vi "06-QNET_MECHKIT_Sonar.vi"() -> ()   [LabVIEW 2017]
doc: "This VI is to be used with the NI-ELVIS and the QNET-Mechatronic Sensors I module. The objective is to calibrate the Sonar sensor."
uses:
  <vilib>/Simulation/Scripting/Companion Diagram/SimConfigNode/SimParams.ctl
  <vilib>/Simulation/Scripting/Companion Diagram/SimConfigNode/_simSolvers.ctl
  <vilib>/Simulation/Implementation/Shared/SIMSCR Execution Mode.ctl
  <vilib>/Simulation/Param Hierarchy/Typedefs/SIMPH Param Control Actions.ctl
  <vilib>/Simulation/Implementation/Shared/NILVSim_ParamChanged.vi
  <vilib>/Simulation/Implementation/Shared/NILVSIM_BeginStep.vi
  <vilib>/DAQmx/read.llb/DAQmx Read.vi
  <vilib>/DAQmx/read.llb/DAQmx Read (Analog DBL 1Chan 1Samp).vi
  <vilib>/Simulation/SignalDisplay/Implementation/NILVSim Time Waveform.llb/SIM Time Waveform (scalar).vi
  <vilib>/Simulation/Utility/Implementation/SIM Halt.vi
  <vilib>/Simulation/Implementation/Shared/NILVSim_Manager.vi
  <vilib>/Utility/error.llb/Clear Errors.vi
  <vilib>/Simulation/Implementation/Shared/NILVSim_FinalizeModel.vi
  <vilib>/Simulation/Implementation/Shared/SIM Unbundle Sim Info.vi
  <vilib>/Simulation/Implementation/Shared/NILVSim_Initialize.vi
  <vilib>/Analysis/6fits.llb/Linear Fit.vi
  <vilib>/DAQmx/miscellaneous.llb/DAQmx Fill In Error Info.vi
  <vilib>/Simulation/Utility/Implementation/NILVSim Get Time and IsAcceptedStep.vi
  <vilib>/Simulation/Implementation/Shared/SIMSH Read Queue.vi
  <vilib>/Simulation/Implementation/Shared/NILVSim_GetModelError.vi
  <vilib>/Simulation/Implementation/Shared/SIM Bundle Sim Info.vi
  <vilib>/Simulation/Scripting/Companion Diagram/SimConfigNode/SimDog.xnode
  <vilib>/Simulation/Implementation/XNodeFramework/SimXNode/SimX.xnode
  <vilib>/Analysis/NI_AALPro.lvlib
  <vilib>/Simulation/Implementation/Shared/NI_SIM_Implementation.lvlib
panel:
  in  "Sampling Rate (Hz)":dbl=100.0 min=0.0 max=1000.0 step=25.0 format="%.1f"
  in  "Device":tag="Dev1"
  in  "Tab Control":enum32{"Collect Data", "Calibrate Sensor"}(tab)
  out "slope":dbl format="%_3f"
  out "intercept":dbl format="%_3f"
  out "Sonar (V)":waveform(dbl)(graph)
  in  "Target Range (in)":dbl[](array[numeric])
  in  "Sensor Measurement (V)":dbl[](array[numeric])
  out "Sensor Readings":T1(graph)
  out "Sonar (inch) 2":dbl(knob) scale=0.0..20.0
  in  "Offset (in)":dbl
  in  "Calibration Gain (in/V)":dbl
  out "Sonar (inch)":waveform(dbl)(graph)
  in  "stop":bool
  # "QNET-MECHKIT Sonar"
  # "NOTE: Place J9 jumper on \"Sonar\" setting."
  # "1) Move target at different positions.\n2) Enter distance between Sonar and target in \"Target Range (in)\" array.\n3) Enter measured sensor values in \"Sensor Measurement (V)\" array."
  # "Linear curve fitting results:"
  # "Enter gain and offset values for sonar to measure the correct target position\n(e.g. display below should read 8-inches when target is 8-inches away from sonar sensor)."
  # "y = Gain*x + Offset\nwhere\nx is the sensor voltage \ny is the output in inches."
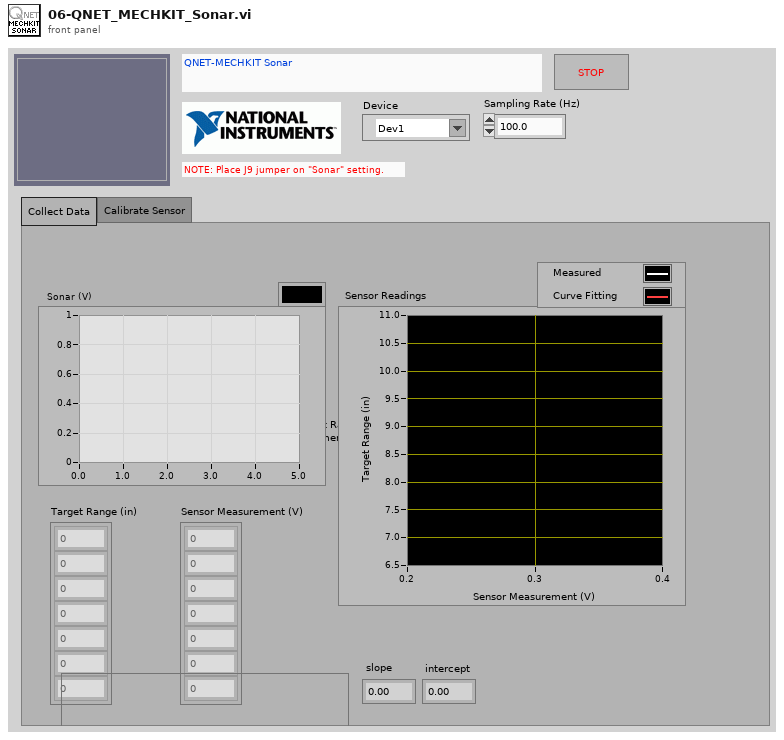
[diagram p1: front panel]
types:
  T1 = cluster{"Sensor Measurement (V)":dbl[], "Best Linear Fit":dbl[]}[]
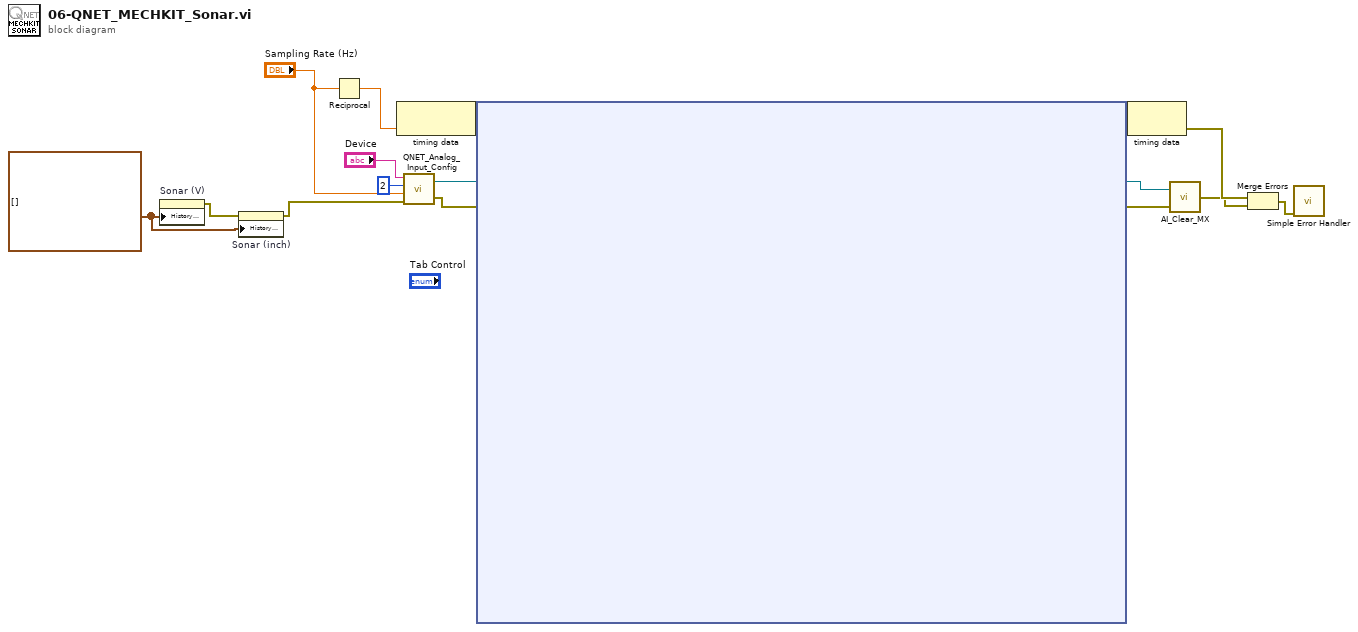
[diagram p0: block diagram]
diagram:
  w1 = waveform(dbl)[] [] ("History Data")
  n1 = property on="Sonar (V)" class="WFChart (strict)"("History Data"=w1) -> (error out=w3:errorcluster)  [unwired: 2 in, 1 out]
  n2 = property on="Sonar (inch)" class="WFChart (strict)"(error in=w3, "History Data"=w1) -> (error out=w2:errorcluster)  [unwired: 1 in, 1 out]
  n3 = Reciprocal(x="Sampling Rate (Hz)") -> (1/x=w8:dbl)
  n4 = node-c288(w8) -> (w16:variant)
  n5 = call "QNET_Analog_Input_Config.vi"("error in"=w2, "sampling rate (Hz)"="Sampling Rate (Hz)", "analog input channel"=u32 2, "dev"="Device") -> ("error out"=w13:errorcluster, "task out"=w12:refnum<k21>)
  n6 = node-c254 ("Simulation Loop")(w16, w13, w12) -> (w15:variant, w11:refnum<k21>, w10:errorcluster)
  n7 = node-c288(w15) -> (w7:errorcluster)
  n8 = call "AI_Clear_MX.vi"("Error in"=w10, "Task in"=w11) -> ("Error out"=w6:errorcluster)
  n9 = Merge Errors(w7, w6) -> (w5:errorcluster)
  n10 = call <vilib>:"Simple Error Handler.vi"("error in (no error)"=w5) -> ()  [unwired: 1 in, 8 out]
